vi "MeasureVoltage.vi"(4 "Device":u8=1, 5 "Serial port":refnum<visa-resource-name>) -> (0 "Voltage":sgl, 1 "Device out":u8=1, 2 "Serial port out":refnum<visa-resource-name>)   [LabVIEW 2021]
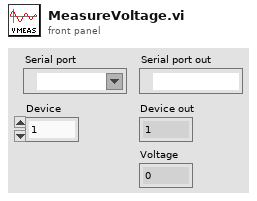
[diagram p1: front panel]
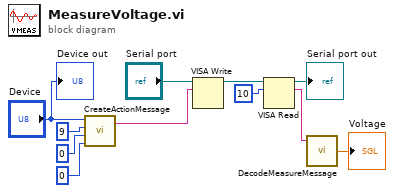
[diagram p0: block diagram]
diagram:
  n1 = call "CreateActionMessage.vi"("Value"=0, "Key"=u32 0, "Action"=u8 9, "Device"="Device") -> ("Message"=w2:string)  [unwired: 1 in]
  n2 = VISA Write(VISA resource name="Serial port", write buffer=w2) -> (VISA resource name out=w11:refnum<visa-resource-name>)  [unwired: 1 in, 2 out]
  n3 = VISA Read(VISA resource name=w11, byte count=u32 10) -> (VISA resource name out=→"Serial port out":refnum<visa-resource-name>, read buffer=w7:string)  [unwired: 1 in, 2 out]
  n4 = call "DecodeMeasureMessage.vi"("Message"=w7) -> ("Voltage"=→"Voltage":sgl)  [unwired: 2 in, 2 out]
  "Device out" <- "Device"
